vi "Segment Valve Time.vi"(11 "Data":string) -> (2 "Cold Segment Valve Time":u16, 3 "Hot Segment Valve Time":u16)   [LabVIEW 2016, in "GEA2_Toolkit.lvlib"]
uses:
  library/GEA2_Toolkit.lvlib
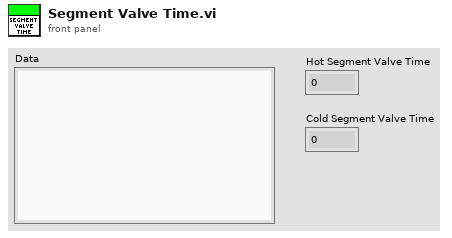
[diagram p1: front panel]
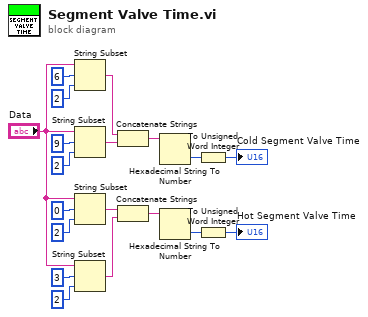
[diagram p0: block diagram]
diagram:
  n1 = String Subset(string="Data", offset (0)=6, length (rest)=2 ("length (rest)")) -> (substring=w10:string)
  n2 = String Subset(string="Data", offset (0)=9, length (rest)=2 ("length (rest)")) -> (substring=w9:string)
  n3 = String Subset(string="Data", offset (0)=0, length (rest)=2 ("length (rest)")) -> (substring=w5:string)
  n4 = String Subset(string="Data", offset (0)=3, length (rest)=2 ("length (rest)")) -> (substring=w6:string)
  n5 = Concatenate Strings(w10, w9) -> (w8:string)
  n6 = Concatenate Strings(w5, w6) -> (w7:string)
  n7 = Hexadecimal String To Number(string=w8) -> (number=w18:u32)  [unwired: 2 in, 1 out]
  n8 = Hexadecimal String To Number(string=w7) -> (number=w16:u32)  [unwired: 2 in, 1 out]
  n9 = To Unsigned Word Integer(number=w18) -> (unsigned 16bit integer=→"Cold Segment Valve Time":u16)
  n10 = To Unsigned Word Integer(number=w16) -> (unsigned 16bit integer=→"Hot Segment Valve Time":u16)
